vi "VS-Compute Vmin,Vmax.vi"(0 "Min":dbl, 5 "Max":dbl, 9 "Scale":T1={"Slope"=0.0, "Offset"=0.0, "Limits"={"Min"=0.0, "Max"=0.0}, "term config"=-1} {"term config" items=["default"=-1, "RSE"=10083, "NRSE"=10078, "Differential"=10106, "Pseudodifferential"=12529]}, 11 "error in (no error)":errorcluster) -> (4 "Vmin":dbl, 6 "Vmax":dbl, 15 "error out":errorcluster)   [LabVIEW 2020]
uses:
  Typedefs/PhysMon-Scale.ctl
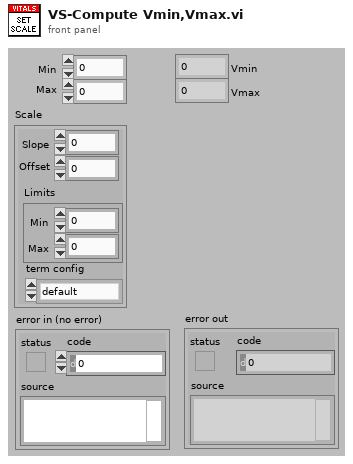
[diagram p1: front panel]
types:
  T1 = typedef "PhysMon-Scale.ctl" = cluster{"Slope":dbl, "Offset":dbl, "Limits":cluster{"Min":dbl, "Max":dbl}, "term config":i32}
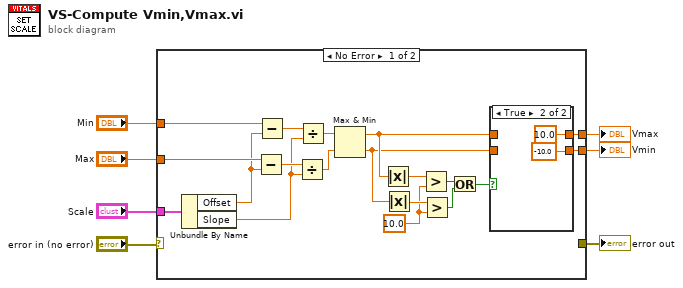
[diagram p0: block diagram]
diagram:
  n1 = case shown="No Error" "error in (no error)" {
    selector: "error in (no error)" -> [_ w31]
    tunnel: [_ w31] -> w6
    tunnel: "Scale" -> [w26 _]
    tunnel: "Max" -> [w25 _]
    tunnel: "Min" -> [w20 _]
    tunnel: [w9 _] -> w2
    tunnel: [w11 _] -> w1
    frame No Error {
      w15 = 10.0 ("y")
      n2 = Unbundle By Name(w26) -> ("Offset"=w21:dbl, "Slope"=w22:dbl)
      n3 = Subtract(x=w25, y=w21) -> (x-y=w24:dbl)
      n4 = Subtract(x=w20, y=w21) -> (x-y=w23:dbl)
      n5 = Divide(x=w24, y=w22) -> (x/y=w18:dbl)
      n6 = Divide(x=w23, y=w22) -> (x/y=w19:dbl)
      n7 = Max & Min(x=w19, y=w18) -> (max(x,y)=w10:dbl, min(x,y)=w8:dbl)
      n8 = Absolute Value(x=w10) -> (abs(x)=w17:dbl)
      n9 = Absolute Value(x=w8) -> (abs(x)=w16:dbl)
      n10 = Greater?(x=w17, y=w15) -> (0:w14:bool)
      n11 = Greater?(x=w16, y=w15) -> (0:w13:bool)
      n12 = Or(x=w14, y=w13) -> (x .or. y?=w12:bool)
      n13 = case shown="True" w12 {
        tunnel: [w28 10.0] -> w11
        tunnel: w10 -> [w28 _]
        tunnel: [w27 -10.0] -> w9
        tunnel: w8 -> [w27 _]
        frame False {
        }
        frame True {
        }
      }
    }
    frame Error {
    }
  }
  "error out" <- w6
  "Vmin" <- w2
  "Vmax" <- w1
